vi "wczytajKrok.vi"(6 "CZUJNIK":u8, 7 "Nr pozycji poziomej":i32, 8 "error in":errorcluster, 9 "Lista punków w poziomie":i32[](array[numeric]), 10 "Kolor czujnika":bool, 11 "LINX Resource in":T1) -> (0 "error out":errorcluster, 1 "Faza ruchu wstępna":T7, 2 "Nowy nr pozycji poziomej":i32, 3 "LINX Resource":T1, 4 "Czy na żądanej pozycji?":bool, 5 "Kolor na czujniku":bool)   [LabVIEW 2014]
uses:
  RuchPoziomy.ctl
  <vilib>/MakerHub/LINX/Private/Type Defs/LINX Ref.ctl
  <vilib>/MakerHub/LINX/Private/Type Defs/Platform.ctl
  <vilib>/MakerHub/LINX/Private/Type Defs/Interface.ctl
  <vilib>/MakerHub/LINX/Private/Device/Type Defs/LINX Device Config.ctl
  <vilib>/MakerHub/LINX/Private/Device/Type Defs/TCP Config.ctl
  <vilib>/MakerHub/LINX/Private/Device/Type Defs/Channels.ctl
  <vilib>/MakerHub/LINX/Public/Peripherals/Digital/Digital Read 1 Chan.vi
  <vilib>/MakerHub/LINX/Public/Peripherals/Digital/Digital Read N Chans.vi
  <vilib>/MakerHub/LINX/Private/Local IO/LinxDigitalRead.vi
  <vilib>/MakerHub/LINX/Public/Utilities/Check Channel.vi
  <vilib>/MakerHub/LINX/Private/Local IO/Handle Errors.vi
  <vilib>/MakerHub/LINX/Private/Utilties/Generate Error.vi
  <vilib>/MakerHub/LINX/LMH-LINX.lvlib
  <vilib>/MakerHub/LINX/Private/Device/Device.lvlib
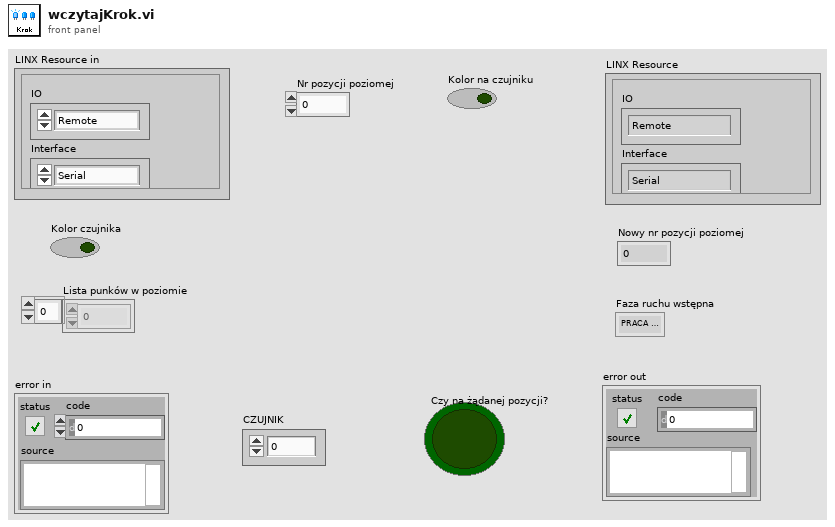
[diagram p1: front panel]
types:
  T1 = typedef "LMH-LINX.lvlib/LINX Ref.ctl" = cluster{"IO":T2, "Interface":T3, "LINX Device Config":T4}
  T2 = typedef "LMH-LINX.lvlib/Platform.ctl" = enum16{"Remote", "Local"}
  T3 = typedef "LMH-LINX.lvlib/Interface.ctl" = enum16{"Serial", "TCP"}
  T4 = typedef "LMH-LINX.lvlib/Device.lvlib/LINX Device Config.ctl" = cluster{"Interface":T3, "COM Port":refnum<visa-resource-name>, "TCP Configuration":T5, "Device Family":u8, "Device ID":u8, "Device Name":string, "TCP Ref":refnum<k5>, "Channels":T6}
  T5 = typedef "LMH-LINX.lvlib/Device.lvlib/TCP Config.ctl" = cluster{"IP Address":string, "Port":u16}
  T6 = typedef "LMH-LINX.lvlib/Channels.ctl" = cluster{"DI":u8[], "DO":u8[], "AI":u8[], "AO":u8[], "PWM":u8[], "QE":u8[], "UART":u8[], "I2C 2":u8[], "SPI":u8[], "CAN":u8[], "Servo":u8[], "AI Ref (V)":dbl, "AI Resolution (Bits)":u8, "AO Ref (V)":dbl, "AO Resolution (Bits)":u8}
  T7 = typedef "RuchPoziomy.ctl" = enum16{"PRACA RĘCZNA", "COFAJ", "NAPRZÓD", "WYŁ."}
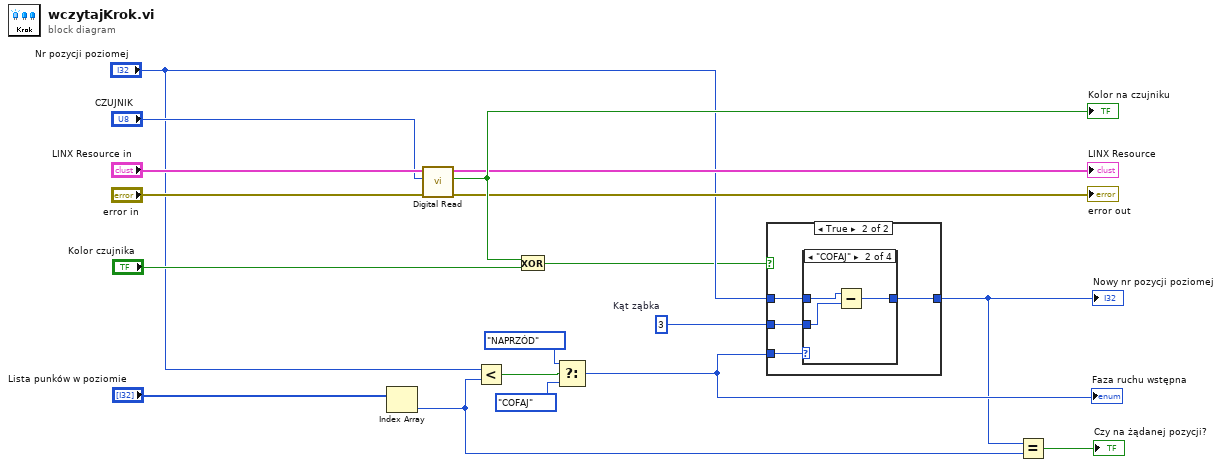
[diagram p0: block diagram]
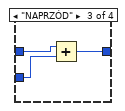
[diagram p4: hidden frame]
diagram:
  w1 = 3  # Kąt ząbka
  n1 = Index Array(array="Lista punków w poziomie") -> (element=w7:i32)  [unwired: 1 in]
  n2 = call-poly <vilib>:"Digital Read.vi"("Error In"="error in", "DI Channel"="CZUJNIK", "LINX Resource"="LINX Resource in") -> ("Error Out"=→"error out":errorcluster, "DI Value"=w14:bool, "LINX Resource"=→"LINX Resource":T1)  [unwired: 6 in]
  "Kolor na czujniku" <- w14
  n3 = Less?(x="Nr pozycji poziomej", y=w7) -> (x < y?=w15:bool)
  n4 = Exclusive Or(1:"Kolor czujnika", 2:w14) -> (0:w2:bool)
  n5 = Select(t=RuchPoziomy."NAPRZÓD" ("Stan poziomy"), s=w15, f=RuchPoziomy."COFAJ" ("Stan poziomy")) -> (s? t:f=w18:T7)
  "Faza ruchu wstępna" <- w18
  n6 = case shown="True" w2 {
    tunnel: "Nr pozycji poziomej" -> [w19 w23]
    tunnel: [w19 w22] -> w8
    tunnel: w18 -> [_ w21]
    tunnel: w1 -> [_ w20]
    frame False {
    }
    frame True {
      n7 = case shown="\"COFAJ\"" w21 {
        tunnel: w23 -> [w24 w26 w29 w31]
        tunnel: [w24 w27 w30 w31] -> w22
        tunnel: w20 -> [_ w25 w28 _]
        frame "PRACA RĘCZNA" {
        }
        frame "COFAJ" {
          n8 = Subtract(x=w26, y=w25) -> (x-y=w27:i32)
        }
        frame "NAPRZÓD" {
          n9 = Add(x=w29, y=w28) -> (x+y=w30:i32)
        }
        frame "WYŁ." {
        }
      }
    }
  }
  "Nowy nr pozycji poziomej" <- w8
  n10 = Equal?(x=w8, y=w7) -> (x = y?=→"Czy na żądanej pozycji?":bool)
